vi "界面UI.vi"() -> ()   [LabVIEW 2016, in "德润超标留样.lvlib"]
uses:
  <vilib>/Utility/miscctls.llb/LVPointTypeDef.ctl
  <vilib>/Utility/config.llb/NI_LVConfig.lvlib
panel:
  out "元素":enum16{"open", "read", "write", "close"}[](array[ring])
  out "队列中元素数量":i32
  in  "时间等比采样":u16=10
  in  "单次采样量":u16=500
  in  "修改门禁密码":bool
  in  "远程复位":bool
  in  "排空当前瓶":bool
  in  "采样方式":enum16{"单采", "双重"}(ring)
  in  "远程留样":bool
  in  "选择留样瓶":bool
  in  "排空留样瓶":bool
  out "采样器状态":T1
  out "Registers":u16[](array[numeric])
  in  "打开串口":bool
  in  "释放串口":bool
  in  "留样模式":T2(ring)=enum."外控留样"
  in  "采样启动":bool
  in  "停止命令":bool
  in  "切换采样器状态":bool
  in  "时间校准":bool
  out "source":string
  out "通讯":bool
  # "只在待机时启动有效"
  # "只在停止时切换有效"
  # "只在待机时启动有效"
  # "只在待机时切换有效"
  # "只在待机时启动有效"
  # "默认：500ml（5-1000）ml （只在停止时写有效）"
  # "默认：10min（2-9999）min （只在停止时写有效）"
  # "德润DR803L超标留样"
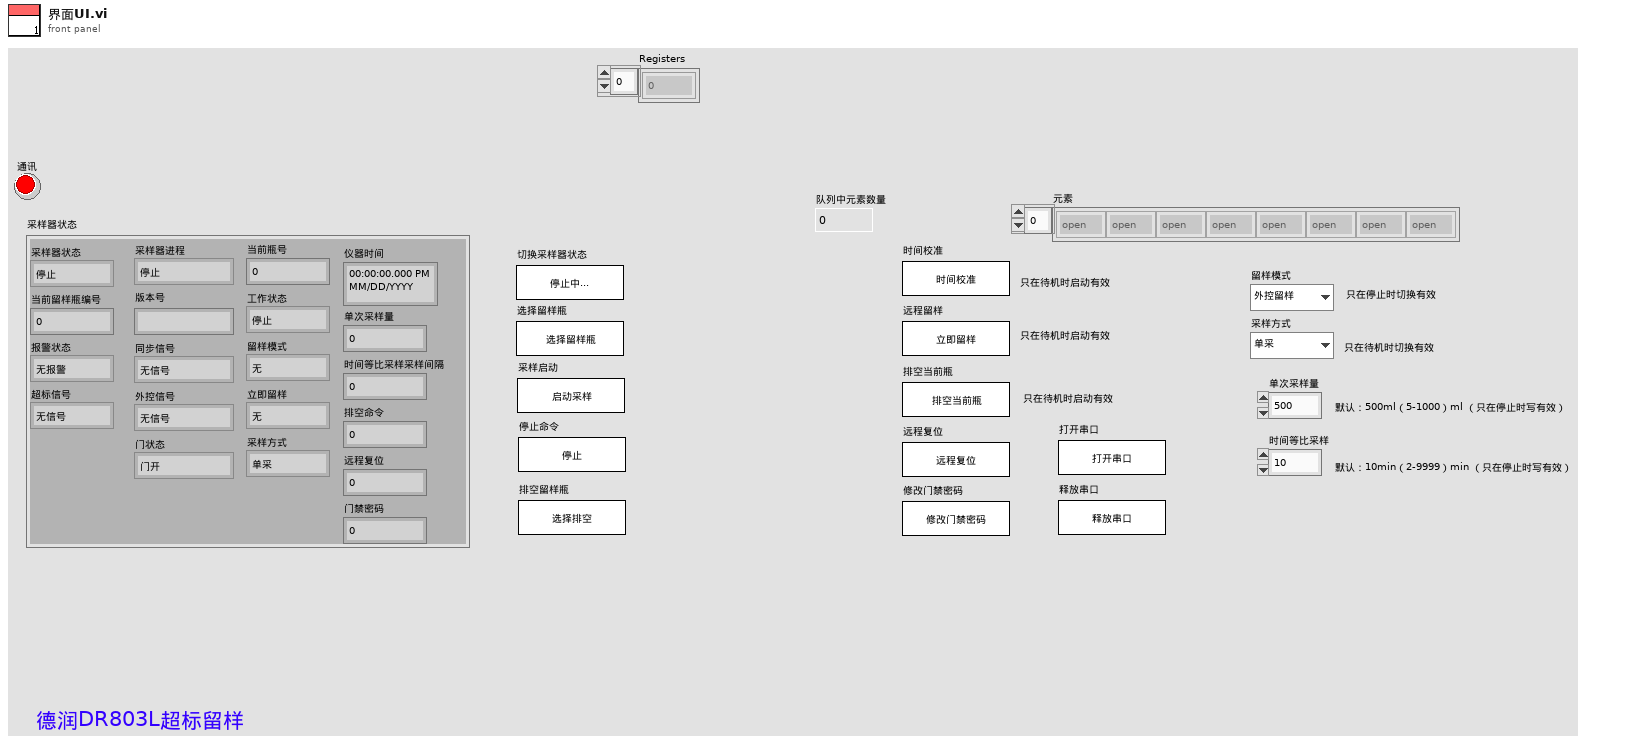
[diagram p1: front panel]
types:
  T1 = cluster{"采样器状态":enum16{"停止", "运行"}, "当前留样瓶编号":u16, "报警状态":enum16{"无报警", "缺水报警"}, "超标信号":enum16{"无信号", "超标信号"}, "采样器进程":enum16{"停止", "待机", "定位校正", "移除瓶盖", "采样瓶排空", "管路润洗", "管存", "进样", "瓶盖密封", "管路排空", "调整采样位置", "采样结束", "采样瓶润洗", "瓶润洗排空"}, "版本号":string, "同步信号":enum16{"无信号", "同步信号"}, "外控信号":enum16{"无信号", "外控信号"}, "门状态":enum16{"门开", "门关"}, "当前瓶号":u16, "工作状态":enum16{"停止", "采样中"}, "留样模式":enum16{"无", "定时留样", "时间等比例", "超标留样", "同步留样", "外控留样"}, "立即留样":enum16{"无", "远程留样"}, "采样方式":enum16{"单采", "双重"}, "仪器时间":timestamp, "单次采样量":u16, "时间等比采样采样间隔":u16, "排空命令":u16, "远程复位":u16, "门禁密码":u16}
  T2 = enum16{"", "定时留样", "时间等比", "超标留样", "同步留样", "外控留样"}
  T3 = cluster{"STEP":enum16{"open", "read", "write", "write single", "close"}, "starting address":u16, "value":u16}
  T4 = typedef "LVPointTypeDef.ctl" = cluster{"Horizontal":i16, "Vertical":i16}
  T5 = typedef "NI_LVConfig.lvlib/Config Data RefNum.ctl" = refnum<k1>
  T6 = enum16{"open", "read", "write", "write single", "close"}
  T7 = typedef "LVDateTimeRec.ctl" = cluster{"秒数的小数部分":dbl, "秒":i32, "分":i32, "时":i32, "日":i32, "月":i32, "年":i32, "天数（周）":i32, "天数（年）":i32, "DST":i32}
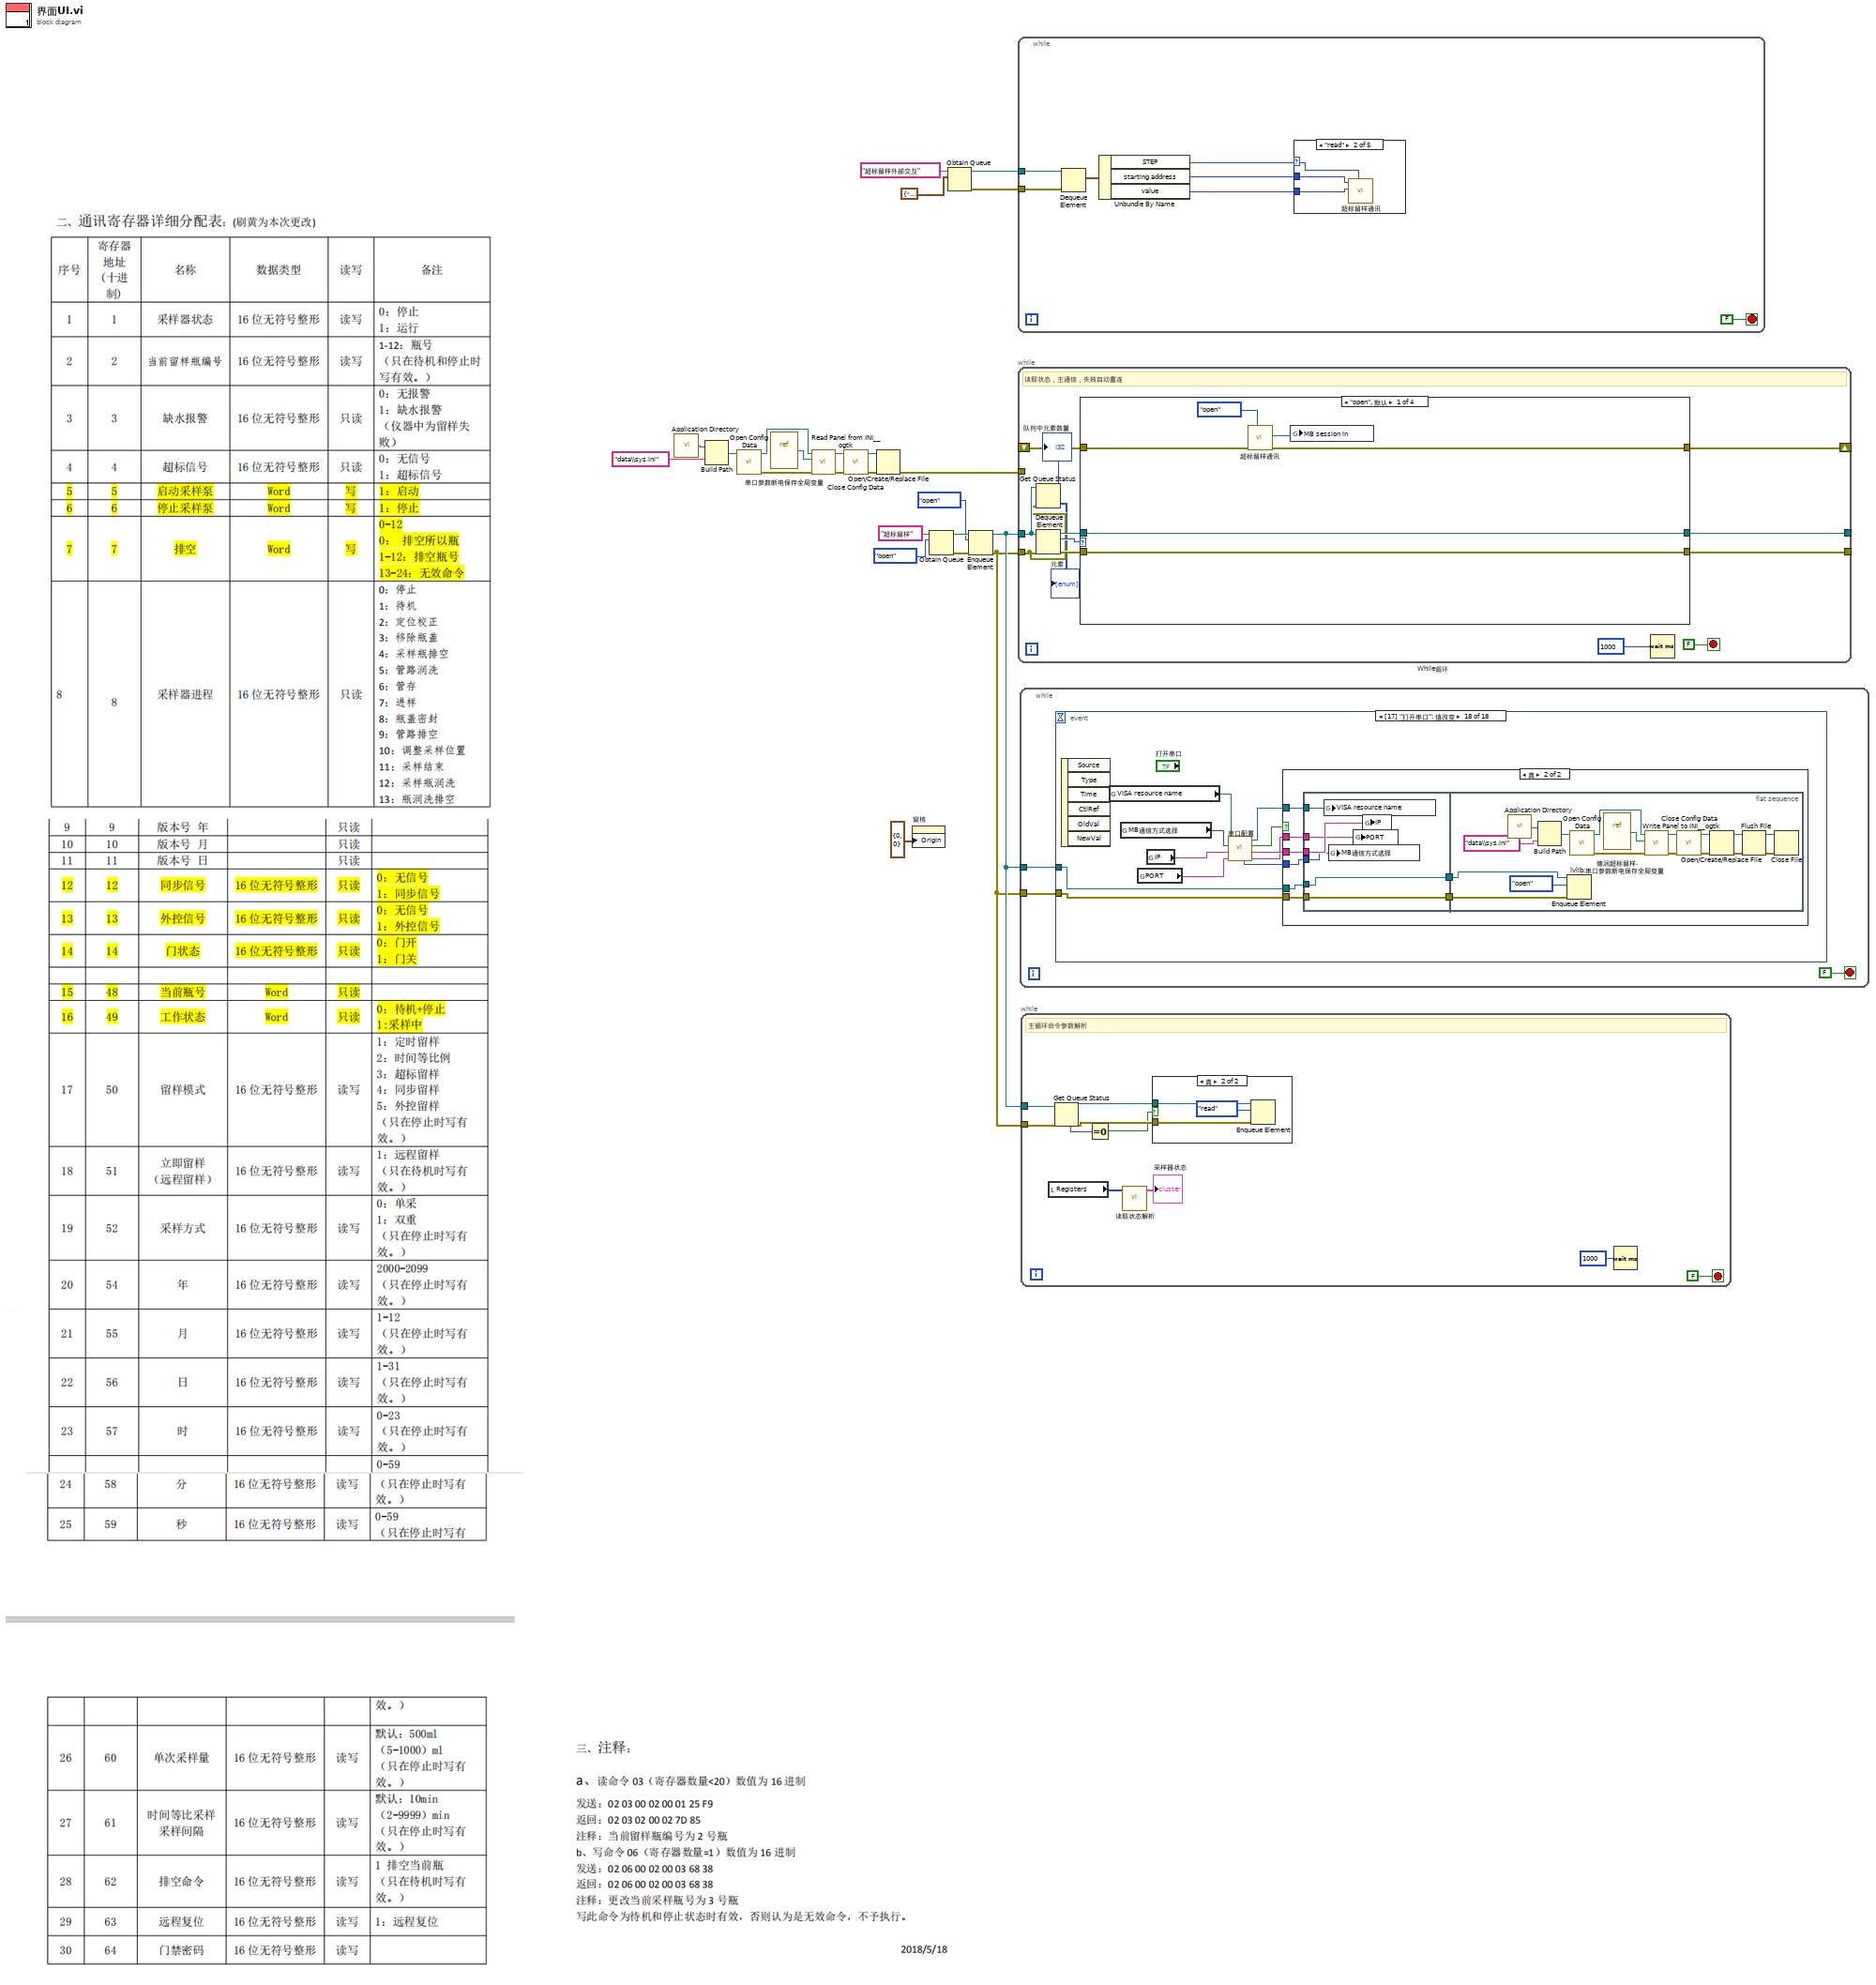
[diagram p0: block diagram]
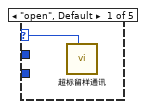
[diagram p2: hidden frame]
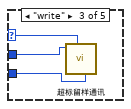
[diagram p3: hidden frame]
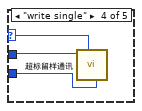
[diagram p4: hidden frame]
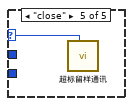
[diagram p5: hidden frame]
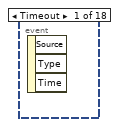
[diagram p6: hidden frame]
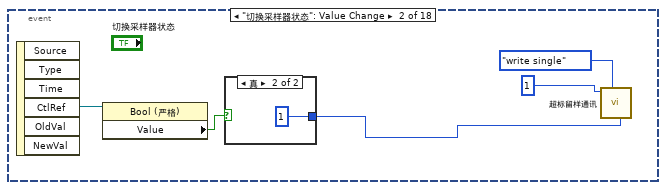
[diagram p7: hidden frame]
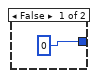
[diagram p8: hidden frame]
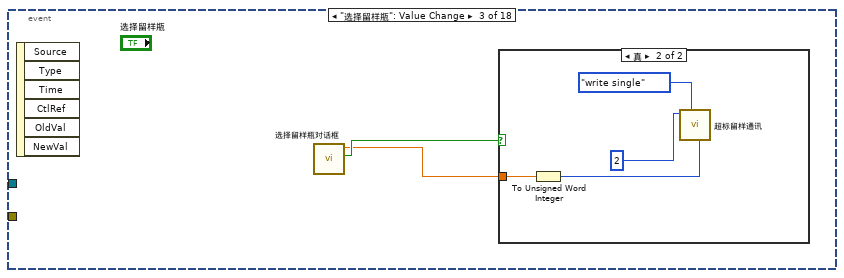
[diagram p9: hidden frame]
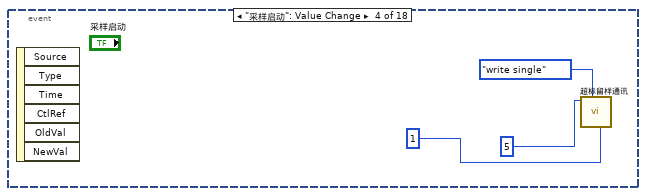
[diagram p11: hidden frame]
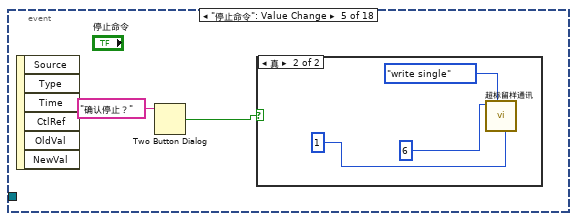
[diagram p12: hidden frame]
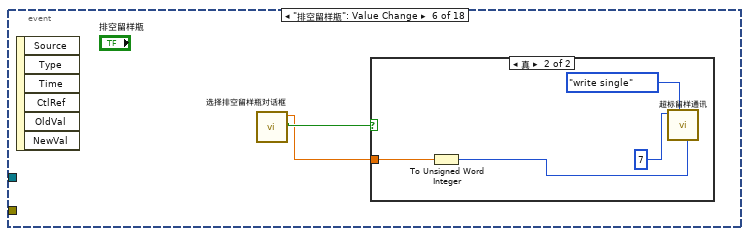
[diagram p14: hidden frame]
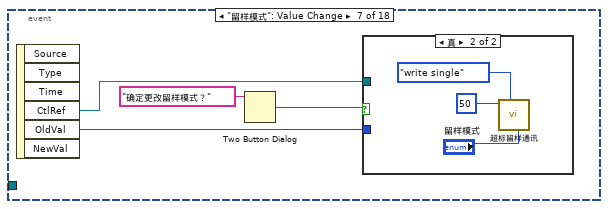
[diagram p16: hidden frame]
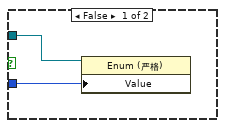
[diagram p17: hidden frame]
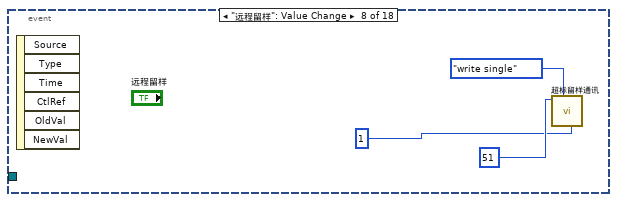
[diagram p18: hidden frame]
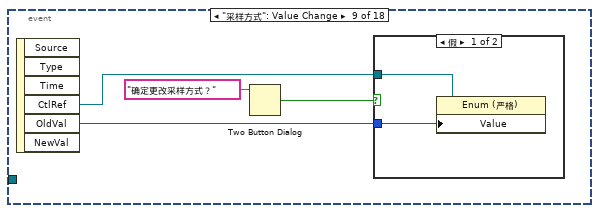
[diagram p19: hidden frame]
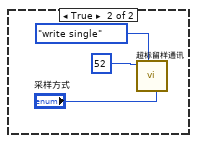
[diagram p20: hidden frame]
diagram:
  n1 = call <vilib>:"Application Directory.vi"() -> ("Application Directory"=w15:path)
  n2 = Build Path(base path=w15, name or relative path="data\\sys.ini" ("名称或相对路径")) -> (appended path=w13:path)
  n3 = call <vilib>:"Open Config Data.vi"("configuration file path"=w13) -> ("error out"=w9:errorcluster, "refnum"=w12:T5)  [unwired: 8 in, 1 out]
  n4 = vi-ref "串口参数断电保存全局变量.vi"() -> (w11:refnum<vi>)
  n5 = call <userlib>:"Read Panel from INI__ogtk.vi"("error in (no error)"=w9, "VI ref"=w11, "refnum"=w12) -> ("error out"=w8:errorcluster, "refnum out"=w10:T5)  [unwired: 7 in]
  n6 = call <vilib>:"Close Config Data.vi"("error in (no error)"=w8, "refnum"=w10) -> ("error out"=w7:errorcluster, "file path"=w6:path)  [unwired: 8 in]
  n7 = Open/Create/Replace File(file path (use dialog)=w6, error in=w7) -> (error out=w5:errorcluster)  [unwired: 4 in, 2 out]
  n8 = property on="窗格" class="Pane"("Origin"=T4 {"Horizontal"=0, "Vertical"=0} ("原点")) -> ()  [unwired: 2 in, 2 out]
  n9 = Obtain Queue(name (unnamed)="超标留样" ("名称（未命名）"), element data type=enum16{"open", "read", "write", "close"}."open") -> (queue out=w21:refnum<queue>, error out=w20:errorcluster)  [unwired: 3 in, 1 out]
  n10 = Obtain Queue(name (unnamed)="超标留样外部交互" ("名称（未命名）"), element data type=T3 {"STEP"=enum."write single", "starting address"=0, "value"=0}) -> (queue out=w2:refnum<queue>, error out=w1:errorcluster)  [unwired: 3 in, 1 out]
  n11 = Enqueue Element(queue=w21, element=enum16{"open", "read", "write", "close"}."open", error in (no error)=w20) -> (queue out=w18:refnum<queue>, error out=w17:errorcluster)  [unwired: 1 in, 1 out]
  n12 = while {
    tunnel: w2 -> [w29]
    tunnel: w1 -> [w28]
    stop <- FALSE stop-if-true
    n13 = Dequeue Element(queue=w29, error in (no error)=w28) -> (element=w27:T3)  [unwired: 1 in, 3 out]
    n14 = Unbundle By Name(w27) -> ("STEP"=w26:T6, "starting address"=w25:u16, "value"=w24:u16)
    n15 = case shown="\"read\"" w26 {
      selector: w26 -> [w31 w34 w37 w40 w41]
      tunnel: w25 -> [_ w33 w36 w39 _]
      tunnel: w24 -> [_ w32 w35 w38 _]
      frame "open", Default {
        n16 = call "超标留样通讯.vi"("STEP"=w31) -> ()  [unwired: 8 in, 3 out]
      }
      frame "read" {
        n17 = call "超标留样通讯.vi"("STEP"=w34, "quantity"=w32, "starting address"=w33) -> ()  [unwired: 6 in, 3 out]
      }
      frame "write" {
        n18 = call "超标留样通讯.vi"("value"=w35, "STEP"=w37, "starting address"=w36) -> ()  [unwired: 6 in, 3 out]
      }
      frame "write single" {
        n19 = call "超标留样通讯.vi"("value"=w38, "STEP"=w40, "starting address"=w39) -> ()  [unwired: 6 in, 3 out]
      }
      frame "close" {
        n20 = call "超标留样通讯.vi"("STEP"=w41) -> ()  [unwired: 8 in, 3 out]
      }
    }
  }
  n21 = while "While循环" {
    tunnel: w18 -> [w45]
    tunnel: w17 -> [w44]
    tunnel: [w49] -> _
    tunnel: [w48] -> _
    shift-right: [w46] -> _
    shift-left: _ -> [w47]
    tunnel: w5 -> [_]
    stop <- FALSE stop-if-true
    # "读取状态，主通信，失败自动重连"
    n22 = Get Queue Status(queue=w45, error in (no error)=w44) -> (# elements in queue=→"队列中元素数量":i32, elements=→"元素":enum16{"open", "read", "write", "close"}[])  [unwired: 1 in, 6 out]
    n23 = Dequeue Element(queue=w45, error in (no error)=w44) -> (queue out=w51:refnum<queue>, element=w52:enum16{"open", "read", "write", "close"}, error out=w50:errorcluster)  [unwired: 1 in, 1 out]
    n24 = case shown="\"open\", 默认" w52 {
      tunnel: [w60 w61 w81 w90] -> w46
      tunnel: w51 -> [w59 w66 w80 w93]
      tunnel: w50 -> [w58 w65 w79 w92]
      tunnel: [w59 w66 w80 w93] -> w49
      tunnel: [w58 w65 w79 w92] -> w48
      tunnel: w47 -> [w57 w71 w83 w94]
      frame "open", Default {
        n25 = call "超标留样通讯.vi"("STEP"=T6."open", "Error in"=w57) -> ("error out"=w60:errorcluster, "MB session in"=w56:refnum<class "MB_Master.lvclass">)  [unwired: 7 in, 1 out]
        n26 = global write "串口参数断电保存全局变量.vi" "MB session in"(w56) -> ()
      }
      frame "read" {
        n27 = call "超标留样通讯.vi"("STEP"=T6."read", "Error in"=w71, "quantity"=u16 70, "starting address"=u16 0) -> ("error out"=w61:errorcluster, "Registers"=w68:u16[])  [unwired: 5 in, 1 out]
        n28 = Unbundle By Name(w61) -> ("status"=w64:bool, "source"=→"source":string)
        n29 = Not(x=w64) -> (.not. x?=→"通讯":bool)
        n30 = case shown="错误" w61 {
          tunnel: w68 -> [w72 _]
          tunnel: w66 -> [_ w77]
          tunnel: w65 -> [_ w76]
          frame No Error {
            "Registers" <- w72
          }
          frame Error {
            n31 = Enqueue Element(queue=w77, element=enum16{"open", "read", "write", "close"}."close" ("元素"), error in (no error)=w76) -> (queue out=w75:refnum<queue>, error out=w74:errorcluster)  [unwired: 1 in, 1 out]
            n32 = Enqueue Element(queue=w75, element=enum16{"open", "read", "write", "close"}."open" ("元素"), error in (no error)=w74) -> ()  [unwired: 1 in, 3 out]
          }
        }
      }
      frame "write" {
        n33 = call "超标留样通讯.vi"("STEP"=T6."write single", "Error in"=w83) -> ("error out"=w81:errorcluster)  [unwired: 7 in, 2 out]
        n34 = case shown="错误" w81 {
          tunnel: w80 -> [_ w85]
          tunnel: w79 -> [_ w84]
          frame No Error {
          }
          frame Error {
            n35 = Enqueue Element(queue=w85, element=enum16{"open", "read", "write", "close"}."close" ("元素"), error in (no error)=w84) -> (queue out=w88:refnum<queue>, error out=w87:errorcluster)  [unwired: 1 in, 1 out]
            n36 = Enqueue Element(queue=w88, element=enum16{"open", "read", "write", "close"}."open" ("元素"), error in (no error)=w87) -> ()  [unwired: 1 in, 3 out]
          }
        }
      }
      frame "close" {
        n37 = call "超标留样通讯.vi"("STEP"=T6."close", "Error in"=w94) -> ("error out"=w90:errorcluster)  [unwired: 7 in, 2 out]
      }
    }
    n38 = Wait (ms)(milliseconds to wait=u32 1000 ("等待时间（毫秒）")) -> ()  [unwired: 1 out]
  }
  n39 = while {
    tunnel: w18 -> [w96]
    tunnel: w17 -> [w95]
    stop <- FALSE stop-if-true
    n40 = event shown="[17] \"打开串口\": 值改变" {
      selector: _ -> [_ _ _ _ _ _ _ _ _ _ _ _ _ _ _ _ _ _]
      dyn-events: _ -> [_ _ _ _ _ _ _ _ _ _ _ _ _ _ _ _ _ _]
      timeout: _ -> [_ _ _ _ _ _ _ _ _ _ _ _ _ _ _ _ _ _]
      tunnel: w96 -> [_ _ _ _ _ _ _ _ _ _ _ _ _ _ _ _ w192 w198]
      tunnel: w95 -> [_ _ _ _ _ _ _ _ _ _ _ _ _ _ _ _ w191 w197]
      event Timeout {
        n41 = event-data() -> ()  [unwired: 1 in, 3 out]
      }
      event "切换采样器状态": Value Change {
        n42 = event-data() -> ("CtlRef"=w102:refnum<vi>)  [unwired: 1 in, 5 out]
        n43 = property class="Bool (严格)"(reference=w102) -> ("Value"=w101:bool)  [unwired: 1 in, 2 out]
        n44 = case shown="真" w101 {
          tunnel: [u16 0 ("索引") u16 1 ("索引")] -> w98
          frame False {
          }
          frame True {
          }
        }
        n45 = call "超标留样通讯.vi"("value"=w98, "STEP"=T6."write single", "starting address"=1 ("索引")) -> ()  [unwired: 6 in, 3 out]
      }
      event "选择留样瓶": Value Change {
        n46 = event-data() -> ()  [unwired: 1 in, 6 out]
        n47 = call "选择留样瓶对话框.vi"() -> ("布尔"=w106:bool, "选择留样瓶"=w105:dbl)  [unwired: 10 in]
        n48 = case shown="真" w106 {
          tunnel: w105 -> [_ w107]
          frame False {
          }
          frame True {
            n49 = To Unsigned Word Integer(number=w107) -> (unsigned 16bit integer=w108:u16)
            n50 = call "超标留样通讯.vi"("value"=w108, "STEP"=T6."write single", "starting address"=2 ("索引")) -> ()  [unwired: 6 in, 3 out]
          }
        }
      }
      event "采样启动": Value Change {
        n51 = event-data() -> ()  [unwired: 1 in, 6 out]
        n52 = call "超标留样通讯.vi"("value"=u16 1 ("新元素/子数组"), "STEP"=T6."write single", "starting address"=5 ("索引")) -> ()  [unwired: 6 in, 3 out]
      }
      event "停止命令": Value Change {
        n53 = event-data() -> ()  [unwired: 1 in, 6 out]
        n54 = Two Button Dialog(message="确认停止？" ("消息")) -> (T button?=w114:bool)  [unwired: 2 in]
        n55 = case shown="真" w114 {
          frame False {
          }
          frame True {
            n56 = call "超标留样通讯.vi"("value"=u16 1 ("新元素/子数组"), "STEP"=T6."write single", "starting address"=6 ("索引")) -> ()  [unwired: 6 in, 3 out]
          }
        }
      }
      event "排空留样瓶": Value Change {
        n57 = event-data() -> ()  [unwired: 1 in, 6 out]
        n58 = call "选择排空留样瓶对话框.vi"() -> ("布尔"=w120:bool, "选择留样瓶"=w119:dbl)  [unwired: 10 in]
        n59 = case shown="真" w120 {
          tunnel: w119 -> [_ w124]
          frame False {
          }
          frame True {
            n60 = To Unsigned Word Integer(number=w124) -> (unsigned 16bit integer=w121:u16)
            n61 = call "超标留样通讯.vi"("value"=w121, "STEP"=T6."write single", "starting address"=7 ("索引")) -> ()  [unwired: 6 in, 3 out]
          }
        }
      }
      event "留样模式": Value Change {
        n62 = event-data() -> ("CtlRef"=w125:refnum<vi>, "OldVal"=w126:T2)  [unwired: 1 in, 4 out]
        n63 = Two Button Dialog(message="确定更改留样模式？" ("消息")) -> (T button?=w127:bool)  [unwired: 2 in]
        n64 = case shown="真" w127 {
          tunnel: w126 -> [w129 _]
          tunnel: w125 -> [w130 _]
          frame False {
            n65 = property class="Enum (严格)"(reference=w130, "Value"=w129) -> ()  [unwired: 1 in, 2 out]
          }
          frame True {
            n66 = call "超标留样通讯.vi"("value"="留样模式", "STEP"=T6."write single", "starting address"=50 ("索引")) -> ()  [unwired: 6 in, 3 out]
          }
        }
      }
      event "远程留样": Value Change {
        n67 = event-data() -> ()  [unwired: 1 in, 6 out]
        n68 = call "超标留样通讯.vi"("value"=u16 1 ("新元素/子数组"), "STEP"=T6."write single", "starting address"=51 ("索引")) -> ()  [unwired: 6 in, 3 out]
      }
      event "采样方式": Value Change {
        n69 = event-data() -> ("CtlRef"=w138:refnum<vi>, "OldVal"=w137:enum16{"单采", "双重"})  [unwired: 1 in, 4 out]
        n70 = Two Button Dialog(message="确定更改采样方式？" ("消息")) -> (T button?=w139:bool)  [unwired: 2 in]
        n71 = case shown="假" w139 {
          tunnel: w138 -> [w142 _]
          tunnel: w137 -> [w141 _]
          frame False {
            n72 = property class="Enum (严格)"(reference=w142, "Value"=w141) -> ()  [unwired: 1 in, 2 out]
          }
          frame True {
            n73 = call "超标留样通讯.vi"("value"="采样方式", "STEP"=T6."write single", "starting address"=52 ("索引")) -> ()  [unwired: 6 in, 3 out]
          }
        }
      }
      event "时间校准": Value Change {
        n74 = event-data() -> ()  [unwired: 1 in, 6 out]
        n75 = Get Date/Time In Seconds() -> (seconds since 1Jan1904=w158:timestamp)
        n76 = Seconds To Date/Time(time stamp (now)=w158) -> (date time rec=w157:T7)  [unwired: 1 in]
        n77 = Unbundle By Name(w157) -> ("年"=w154:i32, "月"=w153:i32, "日"=w152:i32, "时"=w151:i32, "分"=w150:i32, "秒"=w149:i32)
        n78 = Build Array(w154, w153, w152, w151, w150, w149) -> (w148:i32[])
        n79 = Insert Into Array(array=u16[] [] ("values"), new element=w148) -> (w155:u16[])  [unwired: 1 in]
        n80 = call "超标留样通讯.vi"("STEP"=T6."write", "values"=w155, "starting address"=54 ("索引")) -> ()  [unwired: 6 in, 3 out]
      }
      event "单次采样量", "时间等比采样": Mouse Down {
        n81 = event-data() -> ("CtlRef"=w162:refnum<vi>)  [unwired: 1 in, 7 out]
        n82 = property class="DigNum (严格)"(reference=w162) -> (reference out=w161:refnum<vi>, "Value"=w160:u16)  [unwired: 1 in, 1 out]
        n83 = call "数字键盘.vi"("OldNumber"=w160) -> ("NewNumber"=w159:sgl)
        n84 = property class="DigNum (严格)"(reference=w161, "Val(Sgnl)"=w159) -> ()  [unwired: 1 in, 2 out]
      }
      event "单次采样量": Value Change {
        n85 = event-data() -> ()  [unwired: 1 in, 6 out]
        n86 = call "超标留样通讯.vi"("value"="单次采样量", "STEP"=T6."write single", "starting address"=60 ("索引")) -> ()  [unwired: 6 in, 3 out]
      }
      event "时间等比采样": Value Change {
        n87 = event-data() -> ()  [unwired: 1 in, 6 out]
        n88 = call "超标留样通讯.vi"("value"="时间等比采样", "STEP"=T6."write single", "starting address"=61 ("索引")) -> ()  [unwired: 6 in, 3 out]
      }
      event "排空当前瓶": Value Change {
        n89 = event-data() -> ()  [unwired: 1 in, 6 out]
        n90 = Two Button Dialog(message="是否排空当前瓶？" ("消息")) -> (T button?=w169:bool)  [unwired: 2 in]
        n91 = case shown="真" w169 {
          frame False {
          }
          frame True {
            n92 = call "超标留样通讯.vi"("value"=u16 1 ("新元素/子数组"), "STEP"=T6."write single", "starting address"=63 ("索引")) -> ()  [unwired: 6 in, 3 out]
          }
        }
      }
      event "远程复位": Value Change {
        n93 = event-data() -> ()  [unwired: 1 in, 6 out]
        n94 = Two Button Dialog(message="确认复位？" ("消息")) -> (T button?=w174:bool)  [unwired: 2 in]
        n95 = case shown="真" w174 {
          frame False {
          }
          frame True {
            n96 = call "超标留样通讯.vi"("value"=u16 1 ("新元素/子数组"), "STEP"=T6."write single", "starting address"=64 ("索引")) -> ()  [unwired: 6 in, 3 out]
          }
        }
      }
      event "修改门禁密码": Value Change {
        n97 = event-data() -> ()  [unwired: 1 in, 6 out]
        n98 = Two Button Dialog(message="确定修改门禁密码？" ("消息")) -> (T button?=w179:bool)  [unwired: 2 in]
        n99 = case shown="真" w179 {
          frame False {
          }
          frame True {
            n100 = local read "采样器状态"() -> (w182:T1)
            n101 = Unbundle By Name(w182) -> ("门禁密码"=w181:u16)
            n102 = call "数字键盘.vi"("OldNumber"=w181) -> ("NewNumber"=w185:sgl)
            n103 = Less?(x=w185, y=sgl 65535.0) -> (x < y?=w183:bool)
            n104 = case shown="真" w183 {
              tunnel: w185 -> [_ w189]
              frame False {
              }
              frame True {
                n105 = To Unsigned Word Integer(number=w189) -> (unsigned 16bit integer=w186:u16)
                n106 = call "超标留样通讯.vi"("value"=w186, "STEP"=T6."write single", "starting address"=65 ("索引")) -> ()  [unwired: 6 in, 3 out]
              }
            }
          }
        }
      }
      event "释放串口": Value Change {
        n107 = event-data() -> ()  [unwired: 1 in, 6 out]
        n108 = Two Button Dialog(message="确认是否释放串口，释放串口将导致通信失败！" ("消息")) -> (T button?=w190:bool)  [unwired: 2 in]
        n109 = case shown="真" w190 {
          tunnel: w192 -> [_ w195]
          tunnel: w191 -> [_ w194]
          frame False {
          }
          frame True {
            n110 = Enqueue Element(queue=w195, element=enum16{"open", "read", "write", "close"}."close" ("元素"), error in (no error)=w194) -> ()  [unwired: 1 in, 3 out]
          }
        }
      }
      event "打开串口": Value Change {
        n111 = event-data() -> ()  [unwired: 1 in, 6 out]
        n112 = global read "串口参数断电保存全局变量.vi" "VISA resource name"() -> (w206:refnum<visa-resource-name>)
        n113 = global read "串口参数断电保存全局变量.vi" "MB通信方式选择"() -> (w207:enum16{"串口", "TCP"})
        n114 = global read "串口参数断电保存全局变量.vi" "PORT"() -> (w204:string)
        n115 = global read "串口参数断电保存全局变量.vi" "IP"() -> (w205:string)
        n116 = call "串口配置.vi"("PORT"=w204, "IP"=w205, "MB通信方式选择"=w207, "请选择串口:"=w206) -> ("PORT 2"=w200:string, "IP 2"=w201:string, "确认 2"=w203:bool, "VISA资源名称 2"=w202:refnum<visa-resource-name>, "MB通信方式选择 2"=w199:enum16{"串口", "TCP"})  [unwired: 3 in]
        n117 = case shown="真" w203 {
          tunnel: w202 -> [_ w215]
          tunnel: w201 -> [_ w214]
          tunnel: w200 -> [_ w213]
          tunnel: w199 -> [_ w212]
          tunnel: w198 -> [_ w211]
          tunnel: w197 -> [_ w209]
          frame False {
          }
          frame True {
            n118 = flat-sequence {
              tunnel: w215 -> [w221]
              tunnel: w214 -> [w220]
              tunnel: w213 -> [w219]
              tunnel: w212 -> [w218]
              tunnel: w211 -> [w217]
              tunnel: [w217] -> w210
              tunnel: w209 -> [w216]
              tunnel: [w216] -> w208
              tunnel: w210 -> [w223]
              tunnel: w208 -> [w222]
              frame #0 {
                n119 = global write "串口参数断电保存全局变量.vi" "VISA resource name"(w221) -> ()
                n120 = global write "串口参数断电保存全局变量.vi" "MB通信方式选择"(w218) -> ()
                n121 = global write "串口参数断电保存全局变量.vi" "PORT"(w219) -> ()
                n122 = global write "串口参数断电保存全局变量.vi" "IP"(w220) -> ()
              }
              frame #1 {
                n123 = call <vilib>:"Application Directory.vi"() -> ("Application Directory"=w226:path)
                n124 = Build Path(base path=w226, name or relative path="data\\sys.ini" ("名称或相对路径")) -> (appended path=w227:path)
                n125 = Enqueue Element(queue=w223, element=enum16{"open", "read", "write", "close"}."open" ("元素"), error in (no error)=w222) -> ()  [unwired: 1 in, 3 out]
                n126 = call <vilib>:"Open Config Data.vi"("configuration file path"=w227) -> ("error out"=w231:errorcluster, "refnum"=w228:T5)  [unwired: 8 in, 1 out]
                n127 = vi-ref "德润超标留样.lvlib:串口参数断电保存全局变量.vi"() -> (w229:refnum<vi>)
                n128 = call <userlib>:"Write Panel to INI__ogtk.vi"("error in (no error)"=w231, "VI ref"=w229, "refnum"=w228) -> ("error out"=w232:errorcluster, "refnum out"=w230:T5)  [unwired: 7 in]
                n129 = call <vilib>:"Close Config Data.vi"("error in (no error)"=w232, "refnum"=w230) -> ("error out"=w237:errorcluster, "file path"=w238:path)  [unwired: 8 in]
                n130 = Open/Create/Replace File(file path (use dialog)=w238, error in=w237) -> (refnum out=w234:refnum<file>, error out=w233:errorcluster)  [unwired: 4 in, 1 out]
                n131 = Flush File(refnum=w234, error in=w233) -> (refnum out=w235:refnum<file>, error out=w236:errorcluster)
                n132 = Close File(refnum=w235, error in=w236) -> ()  [unwired: 2 out]
              }
            }
          }
        }
      }
    }
  }
  n133 = while {
    tunnel: w18 -> [w246]
    tunnel: w17 -> [w245]
    stop <- FALSE stop-if-true
    # "主循环命令参数解析"
    n134 = local read "Registers"() -> (w240:u16[])
    n135 = Get Queue Status(queue=w246, error in (no error)=w245) -> (queue out=w243:refnum<queue>, error out=w242:errorcluster, # elements in queue=w244:i32)  [unwired: 1 in, 5 out]
    n136 = Equal To 0?(x=w244) -> (x = 0?=w241:bool)
    n137 = call "读取状态解析.vi"("Registers"=w240) -> ("采样器状态"=→"采样器状态":T1)  [unwired: 9 in, 1 out]
    n138 = case shown="真" w241 {
      tunnel: w243 -> [_ w250]
      tunnel: w242 -> [_ w249]
      frame False {
      }
      frame True {
        n139 = Enqueue Element(queue=w250, element=enum16{"open", "read", "write", "close"}."read" ("元素"), error in (no error)=w249) -> ()  [unwired: 1 in, 3 out]
      }
    }
    n140 = Wait (ms)(milliseconds to wait=u32 1000 ("等待时间（毫秒）")) -> ()  [unwired: 1 out]
  }
